vi "Set Customer Work Dispatchers.vi"(8 "error in (no error)":errorcluster, 10 "Customer":refnum<class "Customer.lvclass">, 11 "Coffee Shop In":refnum<class "Coffee Shop.lvclass">) -> (0 "error out":errorcluster, 3 "Coffee Shop Out":refnum<class "Coffee Shop.lvclass">)   [LabVIEW 2020, in "Coffee Shop.lvclass"]
uses:
  Coffee Shop.lvclass
  <vilib>/Astemes/Triarc Framework/Process/Process.lvclass/Process.ctl
  <vilib>/Astemes/Triarc Framework/Process/Public/Lifecycle/Get Lifecycle State.vi
  <vilib>/Astemes/Triarc Framework/Process/Private/SubVIs/Handle Debug Data.vi
  <vilib>/Utility/error.llb/Clear Errors.vi
  <vilib>/Utility/High Resolution Relative Seconds.vi
  <vilib>/Utility/error.llb/Error Cluster From Error Code.vi
  Coffee Shop.lvclass/Coffee Shop.ctl
  <vilib>/Astemes/Triarc Framework/Process/Process.lvclass
  People/Customers/Customer/Customer.lvclass
  C:/Git/astemes-triarc-examples/Coffee Shop/Processes/People/Person/Person.lvclass
  C:/Program Files (x86)/National Instruments/LabVIEW 2020/vi.lib/Astemes/Triarc Framework/View/View.lvclass
  C:/Program Files (x86)/National Instruments/LabVIEW 2020/vi.lib/Astemes/Triarc Framework/Process/Process.lvclass
  C:/Program Files (x86)/National Instruments/LabVIEW 2020/vi.lib/Astemes/Triarc Framework/Base/Base.lvclass
  C:/Program Files (x86)/National Instruments/LabVIEW 2020/vi.lib/Astemes/Triarc Framework/Error Handler Interface/Error Handler Interface.lvclass
  C:/Program Files (x86)/National Instruments/LabVIEW 2020/vi.lib/Astemes/Triarc Framework/Logging/Logging.lvclass
  C:/Git/astemes-triarc-examples/Coffee Shop/Processes/People/Customers/Customer/Customer.lvclass
  C:/Git/astemes-triarc-examples/Coffee Shop/Processes/People/Process Job/Job Handler.lvclass
  C:/Program Files (x86)/National Instruments/LabVIEW 2020/vi.lib/Astemes/Triarc Framework/Async Handler/Async Handler.lvclass
  C:/Program Files (x86)/National Instruments/LabVIEW 2020/vi.lib/Astemes/Triarc Framework/Application/Application.lvclass
  C:/Git/astemes-triarc-examples/Coffee Shop/Processes/Coffee Shop/Coffee Shop.lvclass
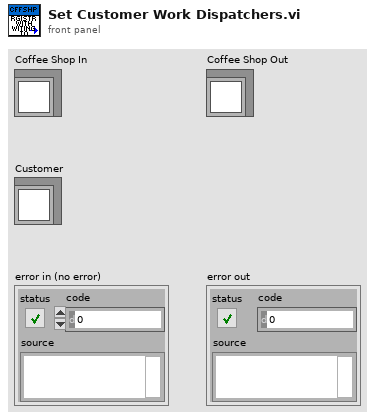
[diagram p1: front panel]
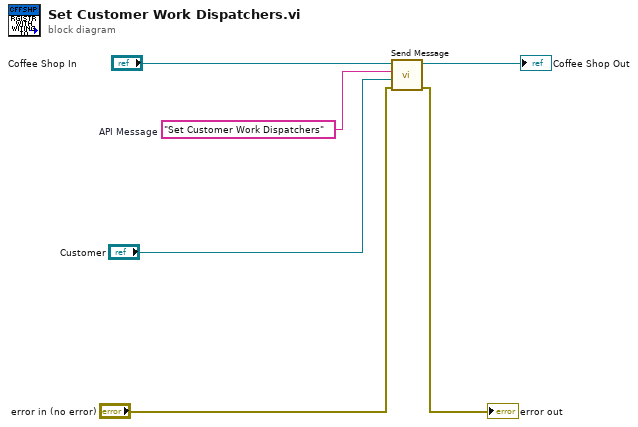
[diagram p0: block diagram]
diagram:
  w3 = "Set Customer Work Dispatchers"  # API Message
  n1 = call <vilib>:"Send Message.vi"("error in (no error)"="error in (no error)", "Message Data"="Customer", "Message"=w3, "Process In"="Coffee Shop In") -> ("error out"=→"error out":errorcluster, "Process Out"=→"Coffee Shop Out":refnum<class "Coffee Shop.lvclass">)  [unwired: 6 in]
